vi "Auto Create String Select Type CaseStructure.vi"(8 "错误输入（无错误）":errorcluster, 11 "FrameNames":string[](array[string])) -> (0 "错误输出":errorcluster)   [LabVIEW 2013]
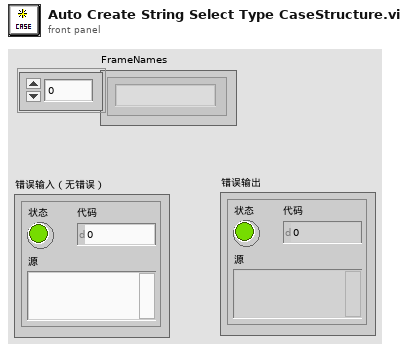
[diagram p1: front panel]
types:
  T1 = cluster{"left":i16, "top":i16, "right":i16, "bottom":i16}
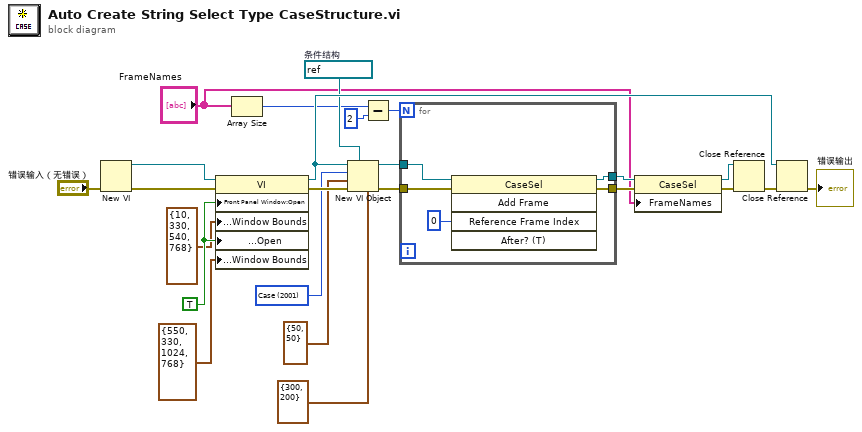
[diagram p0: block diagram]
diagram:
  w20 = refnum<vi> refnum  # 条件结构
  w21 = u32 2001 items=["Absolute Value"=1054, "Access Rights"=1412, "Add"=1050, "Add Array Elements"=1903, "Agitator"=3831, "AllSpoll"=1960, "And"=1061, "And Array Elements"=1911, "Application or VI Refnum"=3412, "Array"=3300, "Array Constant"=2070, "Array Max & Min"=1907, "Array Size"=1809, "Array Subset"=2044, "Array To Cluster"=1168, "Array To Spreadsheet String"=1540, "Array of Strings to Path"=1422, "Atmospheric Tank"=3070, "Automation Close"=8001, "Automation Open"=8000, "Automation RefNum"=3410, "Avogadro Constant (1/mol)"=2030, "Base 10 Logarithm Of e"=2022, "Bin"=3073, "Boolean Array To Number"=1815, "Boolean Constant"=2006, "Boolean To (0,1)"=1167, "Build Array"=2041, "Build Cluster Array"=2047, "Build Path"=1419, "Bundle"=2049, "Bundle By Name"=2057, "Byte Array To String"=1609, "Byte Stream File RefNum"=3408, "Call By Reference Node"=3901, "Call Chain"=1999, "Call Library Function"=2062, "Cancel Button"=3131, "Carriage Return"=2010, "Case"=2001, "Cast Unit Bases"=1079, "Check Valve"=3833, "Checkbox"=3117, "Class Specifier Constant"=2094, "Close Application or VI Reference"=8011, "Close File"=1405, "Cluster"=3400, "Cluster Constant"=2071, "Cluster To Array"=1169, "Code Interface Node"=2050, "Color Box"=3013, "Color Box Constant"=2120, "Color Box Thin Border"=2905, "Color Ramp"=3022, "Combo Box"=3304, "Combo Box Constant"=2088, "Complex Conjugate"=1048, "Complex To Polar"=1045, "Complex To Re/Im"=1044, "Compound Arithmetic"=2200, "Compressor"=3832, "Concatenate Strings"=2040, "Container"=2072, "Control Help Window"=1353, "Control Online Help"=1355, "Convert Unit"=2059, "Conveyer"=3827, "Copy"=1416, "Cosecant"=1204, "Cosine"=1201, "Cotangent"=1205, "Current VI's Menubar"=9000, "Current VI's Path"=1426, "Data Log File RefNum"=3402, "Date/Time To Seconds"=1308, "Decimal Digit?"=1119, "Decimate 1D Array"=2046, "Decrement"=1058, "Default Directory"=1427, "Delete"=1417, "Delete Menu Items"=9004, "DevClear"=1961, "DevClearList"=1962, "Device Control/Status"=1433, "Device RefNum"=3405, "Dial"=3050, "Dialog Button"=3130, "Dialog Checkbox"=3132, "Dialog Radio Button"=3133, "Dialog Recessed Frame"=3624, "Dialog Ring"=3060, "Digital Control"=3000, "Digital Indicator"=3001, "Divide"=1053, "Dlg Numeric"=2100, "Dlg Numeric 2"=3006, "Dlg String"=2110, "Down Arrow"=3824, "Down Bow Valve"=3707, "Down Bow Valve"=3807, "Down Rect Valve"=3806, "Down Rect Valve"=3706, "Down Tee"=3718, "Down Tee"=3818, "EOF"=1410, "Elementary Charge (C)"=2027, "Empty Path"=2033, "Empty String"=2013, "Empty String/Path?"=1112, "Enable Menu Tracking"=9002, "EnableLocal"=1963, "EnableRemote"=1964, "End of Line"=2035, "Enum"=3023, "Enum Constant"=2090, "Equal To 0?"=1113, "Equal?"=1102, "Error Ring"=2039, "Exchanger"=3828, "Exclusive Or"=1063, "Exponential"=1211, "Exponential (Arg) -1"=1222, "File Dialog"=1429, "File Path Control"=3203, "File Path Indicator"=3204, "File/Directory Info"=1413, "FindLstn"=1965, "FindRQS"=1966, "Flat Box"=3602, "Flat Circle"=3605, "Flat Down Triangle"=3623, "Flat Frame"=3608, "Flat Left Triangle"=3620, "Flat Right Triangle"=3621, "Flat Round Button"=3102, "Flat Rounded Box"=3611, "Flat Square Button"=3103, "Flat Up Triangle"=3622, "Flatten To String"=1160, "Flush File"=1406, "For Loop"=2002, "Format & Append"=1512, "Format & Strip"=1534, "Format Date/Time String"=8100, "Format Into String"=2081, "Formula Node"=2004, "Framed Color Box"=3008, "From Decimal"=1184, "From Exponential/Fract/Eng"=1187, "From Hexadecimal"=1185, "From Octal"=1186, "Furnace"=3829, "GPIB Clear"=1954, "GPIB Initialization"=1957, "GPIB Misc"=1956, "GPIB Read"=1951, "GPIB Serial Poll"=1955, "GPIB Status"=1959, "GPIB Trigger"=1953, "GPIB Wait"=1958, "GPIB Write"=1950, "Gauge"=3040, "Generate Occurrence"=1700, "Get Date/Time In Seconds"=1303, "Get Date/Time String"=1600, "Get Help Window Status"=1354, "Get Menu Item Info"=9005, "Get Menu Selection"=9001, "Get Menu Short Cut Info"=9007, "Global Variable"=2060, "Gravitational Constant (N m2/kg2)"=2029, "Greater Or Equal To 0?"=1114, "Greater Or Equal?"=1103, "Greater Than 0?"=1117, "Greater?"=1110, "Handle Peek"=1604, "Handle Poke"=1605, "Hex Digit?"=1123, "HiQ-Script"=9021, "Hopper"=3072, "Horiz Line"=3821, "Horiz Pipe"=3710, "Horiz Pipe"=3810, "Horizontal Fill Slide"=3012, "Horizontal Pointer Slide"=3011, "Horizontal Slide"=3010, "Horizontal Slide Switch"=3114, "Horizontal Switch"=3108, "Horizontal Tank"=3071, "Horizontal Toggle Switch"=3110, "Hyperbolic Cosine"=1215, "Hyperbolic Sine"=1214, "Hyperbolic Tangent"=1216, "IMAQ Session"=3415, "IP to String"=1710, "IVI Delete Session"=8103, "IVI New Session"=8102, "IVI RefNum"=3414, "Implies"=1080, "In Range?"=1127, "Increment"=1057, "Index & Append"=1531, "Index & Bundle Cluster Array"=2056, "Index & Strip"=1532, "Index Array"=2042, "Initialize Array"=2053, "Insert Menu Items"=9003, "Intensity Chart"=3509, "Intensity Graph"=3510, "Interleave 1D Arrays"=2045, "Interpolate 1D Array"=1905, "Inverse Cosine"=1207, "Inverse Hyperbolic Cosine"=1218, "Inverse Hyperbolic Sine"=1217, "Inverse Hyperbolic Tangent"=1219, "Inverse Sine"=1206, "Inverse Tangent"=1208, "Inverse Tangent (2 input)"=1228, "Invoke Node"=3900, "Join Numbers"=1171, "Knob"=3005, "LED Button"=3116, "Lab Gauge"=21009, "Lab Knob"=21000, "Lab Meter"=21008, "Lab Push Button"=21001, "Lab Rocker"=21002, "Lab Tank"=21006, "Lab Thermometer"=21007, "Lab Vertical Toggle Switch"=21005, "Lab Waveform Chart"=21010, "Labeled Oblong Button"=3125, "Labeled Rectangular Button"=3124, "Labeled Round Button"=3122, "Labeled Square Button"=3123, "Left Arrow"=3826, "Left Bow Valve"=3801, "Left Bow Valve"=3701, "Left Down Elbow"=3711, "Left Down Elbow"=3811, "Left Pump"=3713, "Left Pump"=3813, "Left Rect Valve"=3700, "Left Rect Valve"=3800, "Left Tee"=3809, "Left Tee"=3709, "Left Up Elbow"=3708, "Left Up Elbow"=3808, "Less Or Equal To 0?"=1115, "Less Or Equal?"=1104, "Less Than 0?"=1118, "Less?"=1111, "Lexical Class"=1126, "Line Feed"=2011, "List Directory"=1418, "Listbox Symbol Ring"=2038, "Local Variable"=2061, "Lock Range"=1411, "Logarithm Base 10"=1210, "Logarithm Base 2"=1225, "Logarithm Base X"=1224, "Logical Shift"=1081, "MATLAB Script"=9020, "MakeAddr"=1967, "Mantissa & Exponent"=1150, "Match Pattern"=1535, "Max & Min"=1108, "Menu RefNum"=3413, "Menu Ring"=3018, "Menu-Popup Ring"=3017, "Menubar Box"=3627, "Meter"=3030, "Molar Gas Constant (J/(mol K))"=2032, "Motor"=3720, "Motor"=3820, "Move"=1415, "Multiple Selection Listbox"=3208, "Multiple Selection Listbox"=3207, "Multiply"=1052, "Multiply Array Elements"=1904, "Natural Logarithm"=1209, "Natural Logarithm (Arg +1)"=1221, "Natural Logarithm Base"=2020, "Natural Logarithm Of 10"=2023, "Natural Logarithm Of 2"=2024, "Natural Logarithm Of Pi"=2018, "Negate"=1069, "Negative Infinity"=2019, "Network Connection RefNum"=3407, "New Directory"=1402, "New File"=1404, "New VI"=8014, "New VI Object"=8015, "Not"=1064, "Not A Number/Path/Refnum?"=1128, "Not A Path"=2034, "Not And"=1071, "Not Equal To 0?"=1116, "Not Equal?"=1105, "Not Exclusive Or"=1073, "Not Or"=1072, "Not a Refnum"=2036, "Not a Tag"=2037, "Number To Boolean Array"=1814, "Numeric Constant"=2005, "OLE Variant"=3150, "Occurrence RefNum"=3406, "Octal Digit?"=1129, "One Button Dialog"=1340, "Open Application Reference"=8012, "Open Device"=1430, "Open File"=1403, "Open Tank"=3074, "Open VI Object Reference"=8013, "Open VI Reference"=8010, "Or"=1062, "Or Array Elements"=1910, "PPoll"=1969, "PPollConfig"=1970, "PPollUnconfig"=1971, "PassControl"=1968, "Path Constant"=2009, "Path Type"=1421, "Path to Array of Strings"=1423, "Path to String"=1077, "Pi"=2014, "Pi Divided By 2"=2016, "Pi Multiplied By 2"=2015, "Pick Line & Append"=1510, "Pict Ring"=3015, "Picture"=3508, "PixMap"=3505, "PixMap (Do not touch it!!)"=3507, "Planck Constant (J/Hz)"=2026, "Platform Flat Square Button"=3134, "Polar To Complex"=1047, "Positive Infinity"=2025, "Power Of 10"=1212, "Power Of 2"=1223, "Power Of X"=1213, "Pressure Tank"=3075, "Printable?"=1124, "Property Node"=1920, "Pulldown Menu Ring"=3061, "Quit LabVIEW"=1352, "Quotient & Remainder"=1056, "Raised Box"=3600, "Raised Circle"=3603, "Raised Down Triangle"=3615, "Raised Frame"=3606, "Raised Left Triangle"=3612, "Raised Right Triangle"=3613, "Raised Rounded Box"=3609, "Raised Up Triangle"=3614, "Random Number (0-1)"=1070, "RcvRespMsg"=1972, "Re/Im To Complex"=1046, "Read Device"=1432, "Read File"=1407, "ReadStatus"=1973, "Receive"=1974, "ReceiveSetup"=1975, "Recessed Box"=3601, "Recessed Circle"=3604, "Recessed Down Triangle"=3619, "Recessed Frame"=3607, "Recessed Left Triangle"=3616, "Recessed Menu Ring"=3019, "Recessed Right Triangle"=3617, "Recessed Rounded Box"=3610, "Recessed Up Triangle"=3618, "Reciprocal"=1059, "Reciprocal Of Pi"=2017, "Reciprocal Of e"=2021, "Rectangular Stop Button"=3128, "Refnum to Path"=1424, "Refnum to Session"=2306, "Replace Array Element"=2043, "ResetSys"=1976, "Reshape Array"=2055, "Reverse 1D Array"=1900, "Reverse String"=1537, "Right Arrow"=3825, "Right Bow Valve"=3805, "Right Bow Valve"=3705, "Right Down Elbow"=3717, "Right Down Elbow"=3817, "Right Pump"=3819, "Right Pump"=3719, "Right Rect Valve"=3704, "Right Rect Valve"=3804, "Right Tee"=3715, "Right Tee"=3815, "Right Up Elbow"=3814, "Right Up Elbow"=3714, "Ring Constant"=2008, "Rotary Feeder"=3830, "Rotate"=1082, "Rotate 1D Array"=1906, "Rotate Left With Carry"=1606, "Rotate Right With Carry"=1607, "Rotate String"=1536, "Round Button"=3100, "Round LED"=3120, "Round Light"=3104, "Round Push Button"=3112, "Round Push Button 2"=3118, "Round Radio Button"=3106, "Round Stop Button"=3127, "Round To +Infinity"=1076, "Round To -Infinity"=1075, "Round To Nearest"=1055, "Rydberg Constant (/m)"=2031, "Scale By Power Of 2"=1074, "Scan From String"=2080, "Scan String For Tokens"=8101, "Search 1D Array"=1901, "Secant"=1203, "Seconds To Date/Time"=1309, "Seek"=1409, "Select"=1516, "Select & Append"=1511, "Select & Strip"=1533, "Send"=1977, "SendCmds"=1978, "SendDataBytes"=1979, "SendIFC"=1980, "SendLLO"=1982, "SendList"=1981, "SendSetup"=1983, "Sequence"=2000, "Session to Refnum"=2307, "Set Menu Item Info"=9006, "Set Occurrence"=1702, "SetRWLS"=1984, "SetTimeOut"=1985, "Sign"=1049, "Simple Horizontal Slide"=3003, "Simple Numeric"=3029, "Simple Numeric"=2900, "Simple String"=2115, "Simple Vertical Slide"=3002, "Sinc"=1227, "Sine"=1200, "Sine & Cosine"=1220, "Single Selection Listbox"=3206, "Size Handle"=1603, "Sort 1D Array"=1120, "Speed Of Light In Vacuum (m/sec)"=2028, "Split 1D Array"=1908, "Split Number"=1170, "Split String"=1538, "Spreadsheet String To Array"=1539, "Square Button"=3101, "Square LED"=3121, "Square Light"=3105, "Square Push Button"=3113, "Square Push Button 2"=3119, "Square Radio Button"=3107, "Square Root"=1060, "Standard ListBox"=3202, "Stop"=1350, "String Constant"=2007, "String Control"=3200, "String Indicator"=3201, "String Length"=1502, "String Subset"=1503, "String To Byte Array"=1608, "String to IP"=1711, "String to Path"=1078, "String to Tag, String to Tag"=1830, "Strip Path"=1420, "Subtract"=1051, "Swap Bytes"=1162, "Swap Words"=1163, "TCP Close Connection"=1713, "TCP Create Listener"=1717, "TCP Flattened Read"=1718, "TCP Flattened Write"=1719, "TCP Flex Read"=1720, "TCP Flex Write"=1721, "TCP Open Connection"=1715, "TCP Read"=1716, "TCP Wait On Listener"=1712, "TCP Write"=1714, "Tab"=2012, "Table"=3301, "Tag Attribute Ring"=2063, "Tag Constant"=2089, "Tag Control"=3302, "Tag Indicator"=3303, "Tag to String, Tag to String"=1831, "Tangent"=1202, "Tank"=3020, "Temporary Directory"=1435, "TestSRQ"=1986, "TestSys"=1987, "Text & Pict Ring"=3016, "Text Ring"=3014, "Thermometer"=3021, "Threshold 1D Array"=1909, "Tick Count (ms)"=1300, "To Byte Integer"=1140, "To Decimal"=1180, "To Double Precision Complex"=1152, "To Double Precision Float"=1147, "To Engineering"=1183, "To Exponential"=1505, "To Extended Precision Complex"=1154, "To Extended Precision Float"=1149, "To Fractional"=1506, "To G Data"=8003, "To Hexadecimal"=1181, "To Long Integer"=1142, "To Lower Case"=1189, "To OLE Variant"=8002, "To Octal"=1182, "To Quad Integer"=1155, "To Single Precision Complex"=1151, "To Single Precision Float"=1146, "To Unsigned Byte Integer"=1143, "To Unsigned Long Integer"=1145, "To Unsigned Quad Integer"=1156, "To Unsigned Word Integer"=1144, "To Upper Case"=1188, "To Word Integer"=1141, "Transpose 2D Array"=1902, "Trigger"=1988, "TriggerList"=1989, "Two Button Dialog"=1341, "Type Cast"=1166, "Type and Creator"=1434, "UDP Close"=1726, "UDP Open"=1723, "UDP Read"=1724, "UDP Write"=1725, "Unbundle"=2048, "Unbundle By Name"=2058, "Unflatten From String"=1161, "Uniform Dbl Waveform"=3312, "Uniform Int16 Waveform"=3313, "Up Arrow"=3823, "Up Bow Valve"=3803, "Up Bow Valve"=3703, "Up Rect Valve"=3702, "Up Rect Valve"=3802, "Up Tee"=3812, "Up Tee"=3712, "User Item"=3506, "VI Library"=1425, "VISA Assert Trigger"=1929, "VISA Clear"=1927, "VISA Close"=1922, "VISA Disable Event"=1940, "VISA Discard Events"=1941, "VISA Enable Event"=1942, "VISA Find Resource"=1923, "VISA Flush Serial Buffer"=2302, "VISA GPIB Control REN"=2304, "VISA In 16"=1930, "VISA In 32"=1944, "VISA In 8"=1936, "VISA Lock"=1993, "VISA Map Address"=1932, "VISA Mem Alloc"=1997, "VISA Mem Free"=1998, "VISA Move"=2303, "VISA Move In 16"=1948, "VISA Move In 32"=1991, "VISA Move In 8"=1946, "VISA Move Out 16"=1949, "VISA Move Out 32"=1992, "VISA Move Out 8"=1947, "VISA Open"=1921, "VISA Out 16"=1931, "VISA Out 32"=1945, "VISA Out 8"=1937, "VISA Peek 16"=1934, "VISA Peek 32"=1995, "VISA Peek 8"=1938, "VISA Poke 16"=1935, "VISA Poke 32"=1996, "VISA Poke 8"=1939, "VISA Read"=1925, "VISA Read STB"=1928, "VISA Refnum to Session"=2300, "VISA Session"=3409, "VISA Set Serial Buffer Size"=2301, "VISA Status Description"=1924, "VISA Unlock"=1994, "VISA Unmap Address"=1933, "VISA VXI Cmd or Query"=2305, "VISA Wait on Event"=1943, "VISA Write"=1926, "Variant"=3401, "Vert Line"=3822, "Vert Pipe"=3816, "Vert Pipe"=3716, "Vertical Fill Slide"=3009, "Vertical Pointer Slide"=3007, "Vertical Slide"=3004, "Vertical Slide Switch"=3115, "Vertical Switch"=3109, "Vertical Toggle Switch"=3111, "Volume Info"=1414, "Wait (ms)"=1302, "Wait For Activity"=1722, "Wait Until Next ms Multiple"=1327, "Wait for GPIB RQS"=1952, "Wait on Occurrence"=1701, "WaitSRQ"=1990, "Waveform Chart"=3501, "Waveform Graph"=3504, "While Loop"=2003, "White Space?"=1125, "Wire Objects"=8016, "Write Device"=1431, "Write File"=1408, "XY Graph"=3500] ("Object Style")
  w17 = TRUE ("Front Panel Window:Open")
  n1 = New VI(8:"错误输入（无错误）") -> (0:w1:errorcluster, 3:w18:refnum<vi>)  [unwired: 6 out]
  n2 = property class="VI"(reference=w18, error in=w1, "Front Panel Window:Open"=w17, "Front Panel Window:Window Bounds"=T1 {"left"=10, "top"=330, "right"=540, "bottom"=768} ("Block Diagram Window:Window Bounds"), "Block Diagram Window:Open"=w17, "Block Diagram Window:Window Bounds"=T1 {"left"=550, "top"=330, "right"=1024, "bottom"=768}) -> (reference out=w22:refnum<vi>, error out=w23:errorcluster)
  n3 = Array Size(array="FrameNames") -> (size(s)=w6:i32)
  n4 = New VI Object(vi object class=w20, owner refnum=w22, style=w21, position/next to=cluster{"Horizontal":i16, "Vertical":i16} {"Horizontal"=50, "Vertical"=50}, 4:cluster{"Width":u32, "Height":u32} {"Width"=300, "Height"=200} ("bounds"), 8:w23) -> (object refnum=w9:refnum<vi>, 0:w8:errorcluster)  [unwired: 1 in, 1 out]
  n5 = Subtract(x=w6, y=2) -> (x-y=w4:i32)
  n6 = for {
    N: w4 -> [_]
    tunnel: [w28] -> w14
    tunnel: [w27] -> w13
    tunnel: w9 -> [w26]
    tunnel: w8 -> [w25]
    n7 = invoke class="CaseSel" method="Add Frame"(reference=w26, error in=w25, "Reference Frame Index"=u32 0 ("参考帧索引")) -> (reference out=w28:refnum<vi>, error out=w27:errorcluster)  [unwired: 2 in, 3 out]
  }
  n8 = property class="CaseSel"(reference=w14, error in=w13, "FrameNames"="FrameNames") -> (reference out=w12:refnum<vi>, error out=w11:errorcluster)
  n9 = Close Reference(reference=w12, error in (no error)=w11) -> (error out=w10:errorcluster)
  n10 = Close Reference(reference=w22, error in (no error)=w10) -> (error out=→"错误输出":errorcluster)
